vi "Helmholtz2D_Solver.vi"(0 "F(x, y)":dbl[][](array[numeric]), 5 "k":dbl=1.0, 7 "a":dbl, 9 "Domain":T2={"x"={"start x"=0.0, "end x"=1.0, "# of x-points"=11}, "y"={"start y"=0.0, "end y"=1.0, "# of y-points"=11}}, 11 "error in (no error)":errorcluster, 12 "Boundary Condition":cluster{"type":T1, "Value":dbl[]}[](array[cluster]) {"type" items=["Dirichlet", "Neumann"]}) -> (4 "U(x, y)":dbl[][](array[numeric]), 15 "error out":errorcluster)   [LabVIEW 2017, in "NI_PDE.lvlib"]
uses:
  <vilib>/gmath/NI_PDE.lvlib
  <vilib>/gmath/pde.llb/Common/PDE_BC Type.ctl
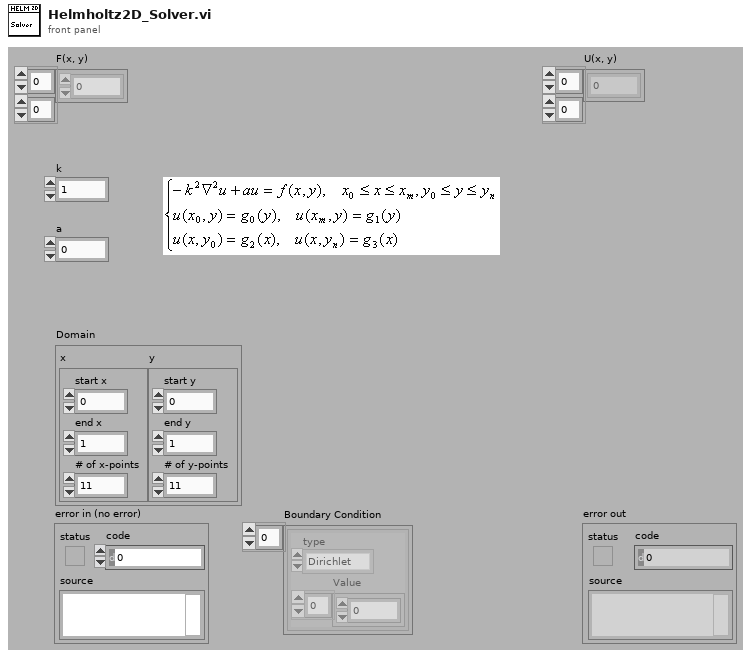
[diagram p1: front panel]
types:
  T1 = typedef "NI_PDE.lvlib/PDE_BC Type.ctl" = i32
  T2 = cluster{"x":cluster{"start x":dbl, "end x":dbl, "# of x-points":i32}, "y":cluster{"start y":dbl, "end y":dbl, "# of y-points":i32}}
  T3 = typedef "NI_Matrix.lvlib/RealMatrix.ctl" = dbl[][]
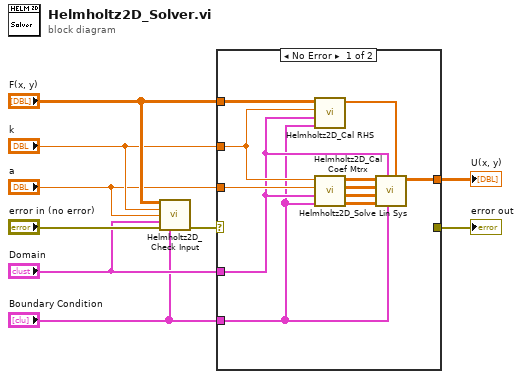
[diagram p0: block diagram]
diagram:
  n1 = call <vilib>:"Helmholtz2D_Check Input.vi"("F(x, y)"="F(x, y)", "k"="k", "a"="a", "Domain"="Domain", "error in (no error)"="error in (no error)", "Boundary Condition"="Boundary Condition") -> ("error out"=w8:errorcluster)  [unwired: 9 out]
  n2 = case shown="No Error" w8 {
    selector: w8 -> [_ w21]
    tunnel: "F(x, y)" -> [w20 _]
    tunnel: "k" -> [w19 _]
    tunnel: "a" -> [w18 _]
    tunnel: "Domain" -> [w13 _]
    tunnel: "Boundary Condition" -> [w12 _]
    tunnel: [_ w21] -> w2
    tunnel: [w10 _] -> w1
    frame No Error {
      n3 = call <vilib>:"Helmholtz2D_Cal RHS.vi"("Boundary Condition"=w12, "Domain"=w13, "k"=w19, "F(x, y)"=w20) -> ("RHS"=w11:dbl[])  [unwired: 7 out]
      n4 = call <vilib>:"Helmholtz2D_Cal Coef Mtrx.vi"("Boundary Condition"=w12, "Domain"=w13, "a"=w18, "k"=w19) -> ("D"=w14:T3, "C"=w15:T3, "D'"=w16:T3, "C'"=w17:T3)  [unwired: 4 out]
      n5 = call <vilib>:"Helmholtz2D_Solve Lin Sys.vi"("RHS"=w11, "Boundary Condition"=w12, "Domain"=w13, "D"=w14, "C"=w15, "D'"=w16, "C'"=w17) -> ("U(x, y)"=w10:dbl[][])  [unwired: 4 out]
    }
    frame Error {
    }
  }
  "U(x, y)" <- w1
  "error out" <- w2
